vi "Test Uninitialised Singleton.vi"(11 "Test Case In":refnum<class "Singleton.lvclass">) -> (0 "error out":errorcluster, 3 "Test Case Out":refnum<class "Singleton.lvclass">)   [LabVIEW 2020, in "Singleton.lvclass"]
uses:
  Singleton.lvclass
  C:/Program Files/National Instruments/LabVIEW 2025/vi.lib/Astemes/LUnit/Test Case.lvclass
  <vilib>/Astemes/LUnit/Test Case.lvclass/Test Case.ctl
  <vilib>/Comparison/Equal/Equal Functor/Equal Functor.lvclass
  Singleton.lvclass/Singleton.ctl
  Source/Singleton/Singleton.lvlib
  <vilib>/Astemes/LUnit/Palette/Advanced Assertions/LUnit Advanced Assertions.lvlib
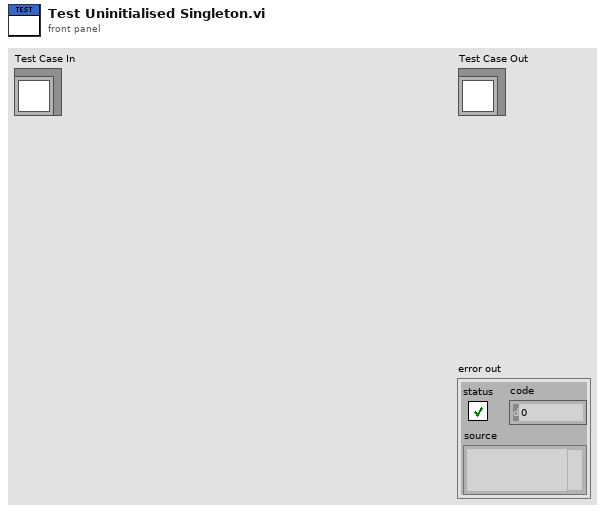
[diagram p1: front panel]
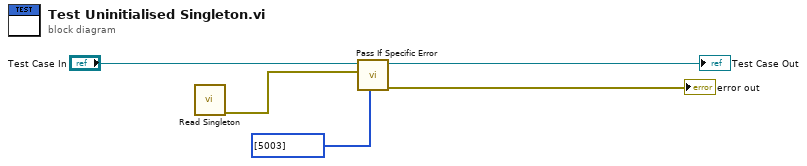
[diagram p0: block diagram]
diagram:
  n1 = call "Read Singleton.vi"() -> ("error out"=w5:errorcluster)  [unwired: 10 in, 1 out]
  n2 = call <vilib>:"Pass If Specific Error.vi"("Error Codes"=i32[] [5003], "Assert error"=w5, "LUnit Test Case In"="Test Case In") -> ("error out"=→"error out":errorcluster, "LUnit Test Case Out"=→"Test Case Out":refnum<class "Singleton.lvclass">)  [unwired: 7 in]
